vi "Create Frame (graphic).vi"(6 "stylename":string, 8 "error in (no error)":errorcluster, 9 "drawName":string, 10 "Graphic file":path, 11 "ooWriter in":refnum<class "ooCalc.lvclass">) -> (0 "error out":errorcluster, 2 "Frame (graphic)":refnum<k24>, 3 "ooWriter out":refnum<class "ooCalc.lvclass">)   [LabVIEW 2009, in "ooCalc.lvclass"]
uses:
  ooCalc.lvclass
  C:/Projets/LAVAG/OpenOfficeRGT/AODL/DLLs/AODL.dll
  ooCalc.lvclass/ooCalc.ctl
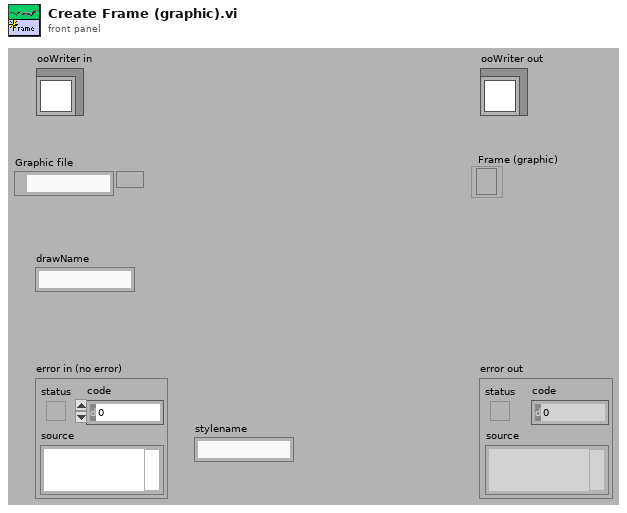
[diagram p1: front panel]
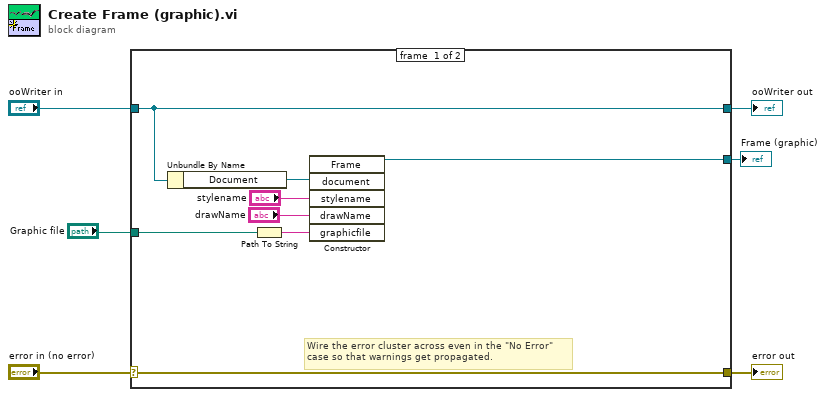
[diagram p0: block diagram]
diagram:
  n1 = case shown="No Error" "error in (no error)" {
    selector: "error in (no error)" -> [w14 w16]
    tunnel: [w14 w16] -> w5
    tunnel: [w13 w15] -> w3
    tunnel: "ooWriter in" -> [w13 w15]
    tunnel: "Graphic file" -> [w11 _]
    tunnel: [w7 _] -> w1
    frame #0 {
      # "Wire the error cluster across even in the \"No Error\"\ncase so that warnings get propagated."
      n2 = Unbundle By Name(w13) -> ("Document"=w12:refnum<k24>)
      n3 = Path To String(path=w11) -> (string=w10:string)
      n4 = constructor class="Frame"("document"=w12, "stylename"="stylename", "drawName"="drawName", "graphicfile"=w10) -> (reference out=w7:refnum<k24>)  [unwired: 3 in, 6 out]
    }
    frame #1 {
    }
  }
  "error out" <- w5
  "ooWriter out" <- w3
  "Frame (graphic)" <- w1
